vi "initialization.vi"(9 "软件版本":refnum<vi>, 10 "updateconfiguration":refnum<vi>) -> ()   [LabVIEW 2016, in "数据传输系统.lvlib"]
uses:
  <vilib>/Utility/config.llb/Read Key (String).vi
  <vilib>/Utility/config.llb/NI_LVConfig.lvlib
panel:
  in  "参数数值":T1={"CODMn"=TRUE, "CODCr"=TRUE, "DO"=TRUE, "铜"=TRUE, "PH"=TRUE, "氨氮"=TRUE, "比电导率"=TRUE, "水温"=TRUE, "COD"=TRUE, "浊度"=TRUE, "总氮"=TRUE, "总磷"=TRUE, "叶绿素a"=TRUE, "藻密度"=TRUE, "水位"=TRUE, "流速"=TRUE, "瞬时流量"=TRUE, "累积流量"=TRUE, "亚硝氮"=TRUE, "硫化物"=TRUE, "ORP"=TRUE, "铅"=TRUE, "镉"=TRUE, "锌"=TRUE, "镍"=TRUE, "锰"=TRUE, "汞"=TRUE, "气温"=TRUE, "气压"=TRUE, "风速"=TRUE, "风向"=TRUE, "盐度"=TRUE, "磷酸盐"=TRUE, "硝氮"=TRUE, "氟化物"=TRUE}
  out "配置表格":string[][](table)
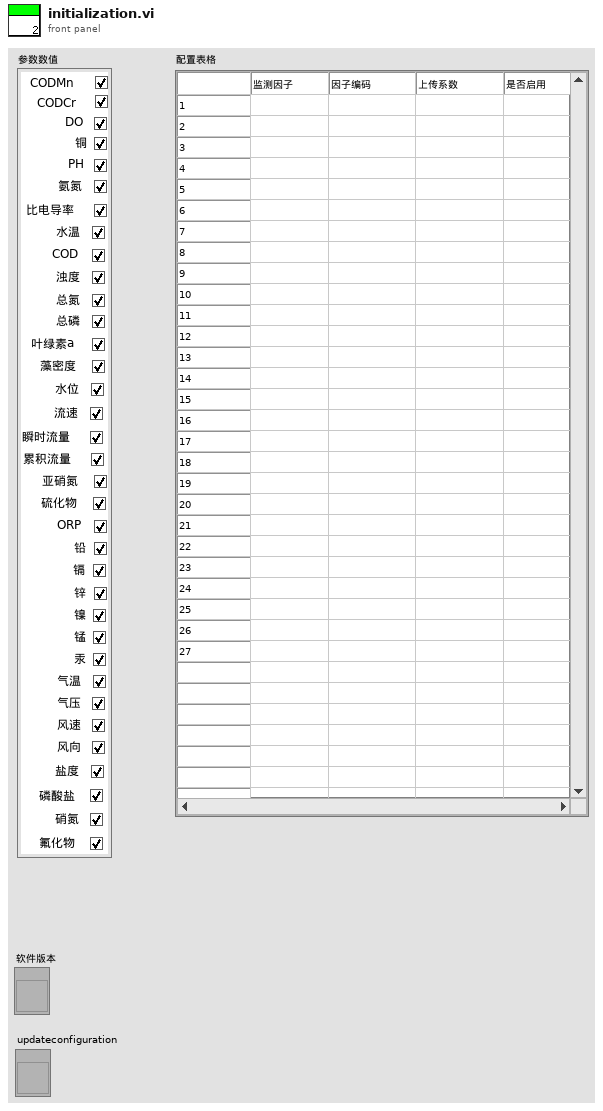
[diagram p1: front panel]
types:
  T1 = cluster{"CODMn":bool, "CODCr":bool, "DO":bool, "铜":bool, "PH":bool, "氨氮":bool, "比电导率":bool, "水温":bool, "COD":bool, "浊度":bool, "总氮":bool, "总磷":bool, "叶绿素a":bool, "藻密度":bool, "水位":bool, "流速":bool, "瞬时流量":bool, "累积流量":bool, "亚硝氮":bool, "硫化物":bool, "ORP":bool, "铅":bool, "镉":bool, "锌":bool, "镍":bool, "锰":bool, "汞":bool, "气温":bool, "气压":bool, "风速":bool, "风向":bool, "盐度":bool, "磷酸盐":bool, "硝氮":bool, "氟化物":bool}
  T2 = cluster{"setini":string, "sysini":string, "hechaini":string, "actualwrite":string, "actualread":string, "datasent":string, "反控命令信息队列":string, "反控与仪器交互":string}
  T3 = cluster{"CODMn":string, "CODCr":string, "DO":string, "铜":string, "PH":string, "氨氮":string, "比电导率":string, "水温":string, "COD":string, "浊度":string, "总氮":string, "总磷":string, "叶绿素a":string, "藻密度":string, "水位":string, "流速":string, "瞬时流量":string, "累积流量":string, "亚硝酸盐":string, "硫化物":string, "ORP":string, "铅":string, "镉":string, "锌":string, "镍":string, "锰":string, "汞":string, "气温":string, "气压":string, "风速":string, "风向":string, "盐度":string, "磷酸盐":string, "硝氮":string, "氟化物":string}
  T4 = typedef "NI_LVConfig.lvlib/Config Data RefNum.ctl" = refnum<k1>
  T5 = cluster{"[0]":string, "[1]":string, "[2]":string, "[3]":string, "[4]":string, "[5]":string, "[6]":string, "[7]":string, "[8]":string, "[9]":string, "[10]":string, "[11]":string, "[12]":string, "[13]":string, "[14]":string, "[15]":string, "[16]":string, "[17]":string, "[18]":string, "[19]":string, "[20]":string, "[21]":string, "[22]":string, "[23]":string, "[24]":string, "[25]":string, "[26]":string, "[27]":string, "[28]":string, "[29]":string, "[30]":string, "[31]":string, "[32]":string, "[33]":string, "[34]":string}
  T6 = cluster{"主机":string, "用户":string, "密码":string, "远程路径":string, "下载文件名":string, "软件版本":string}
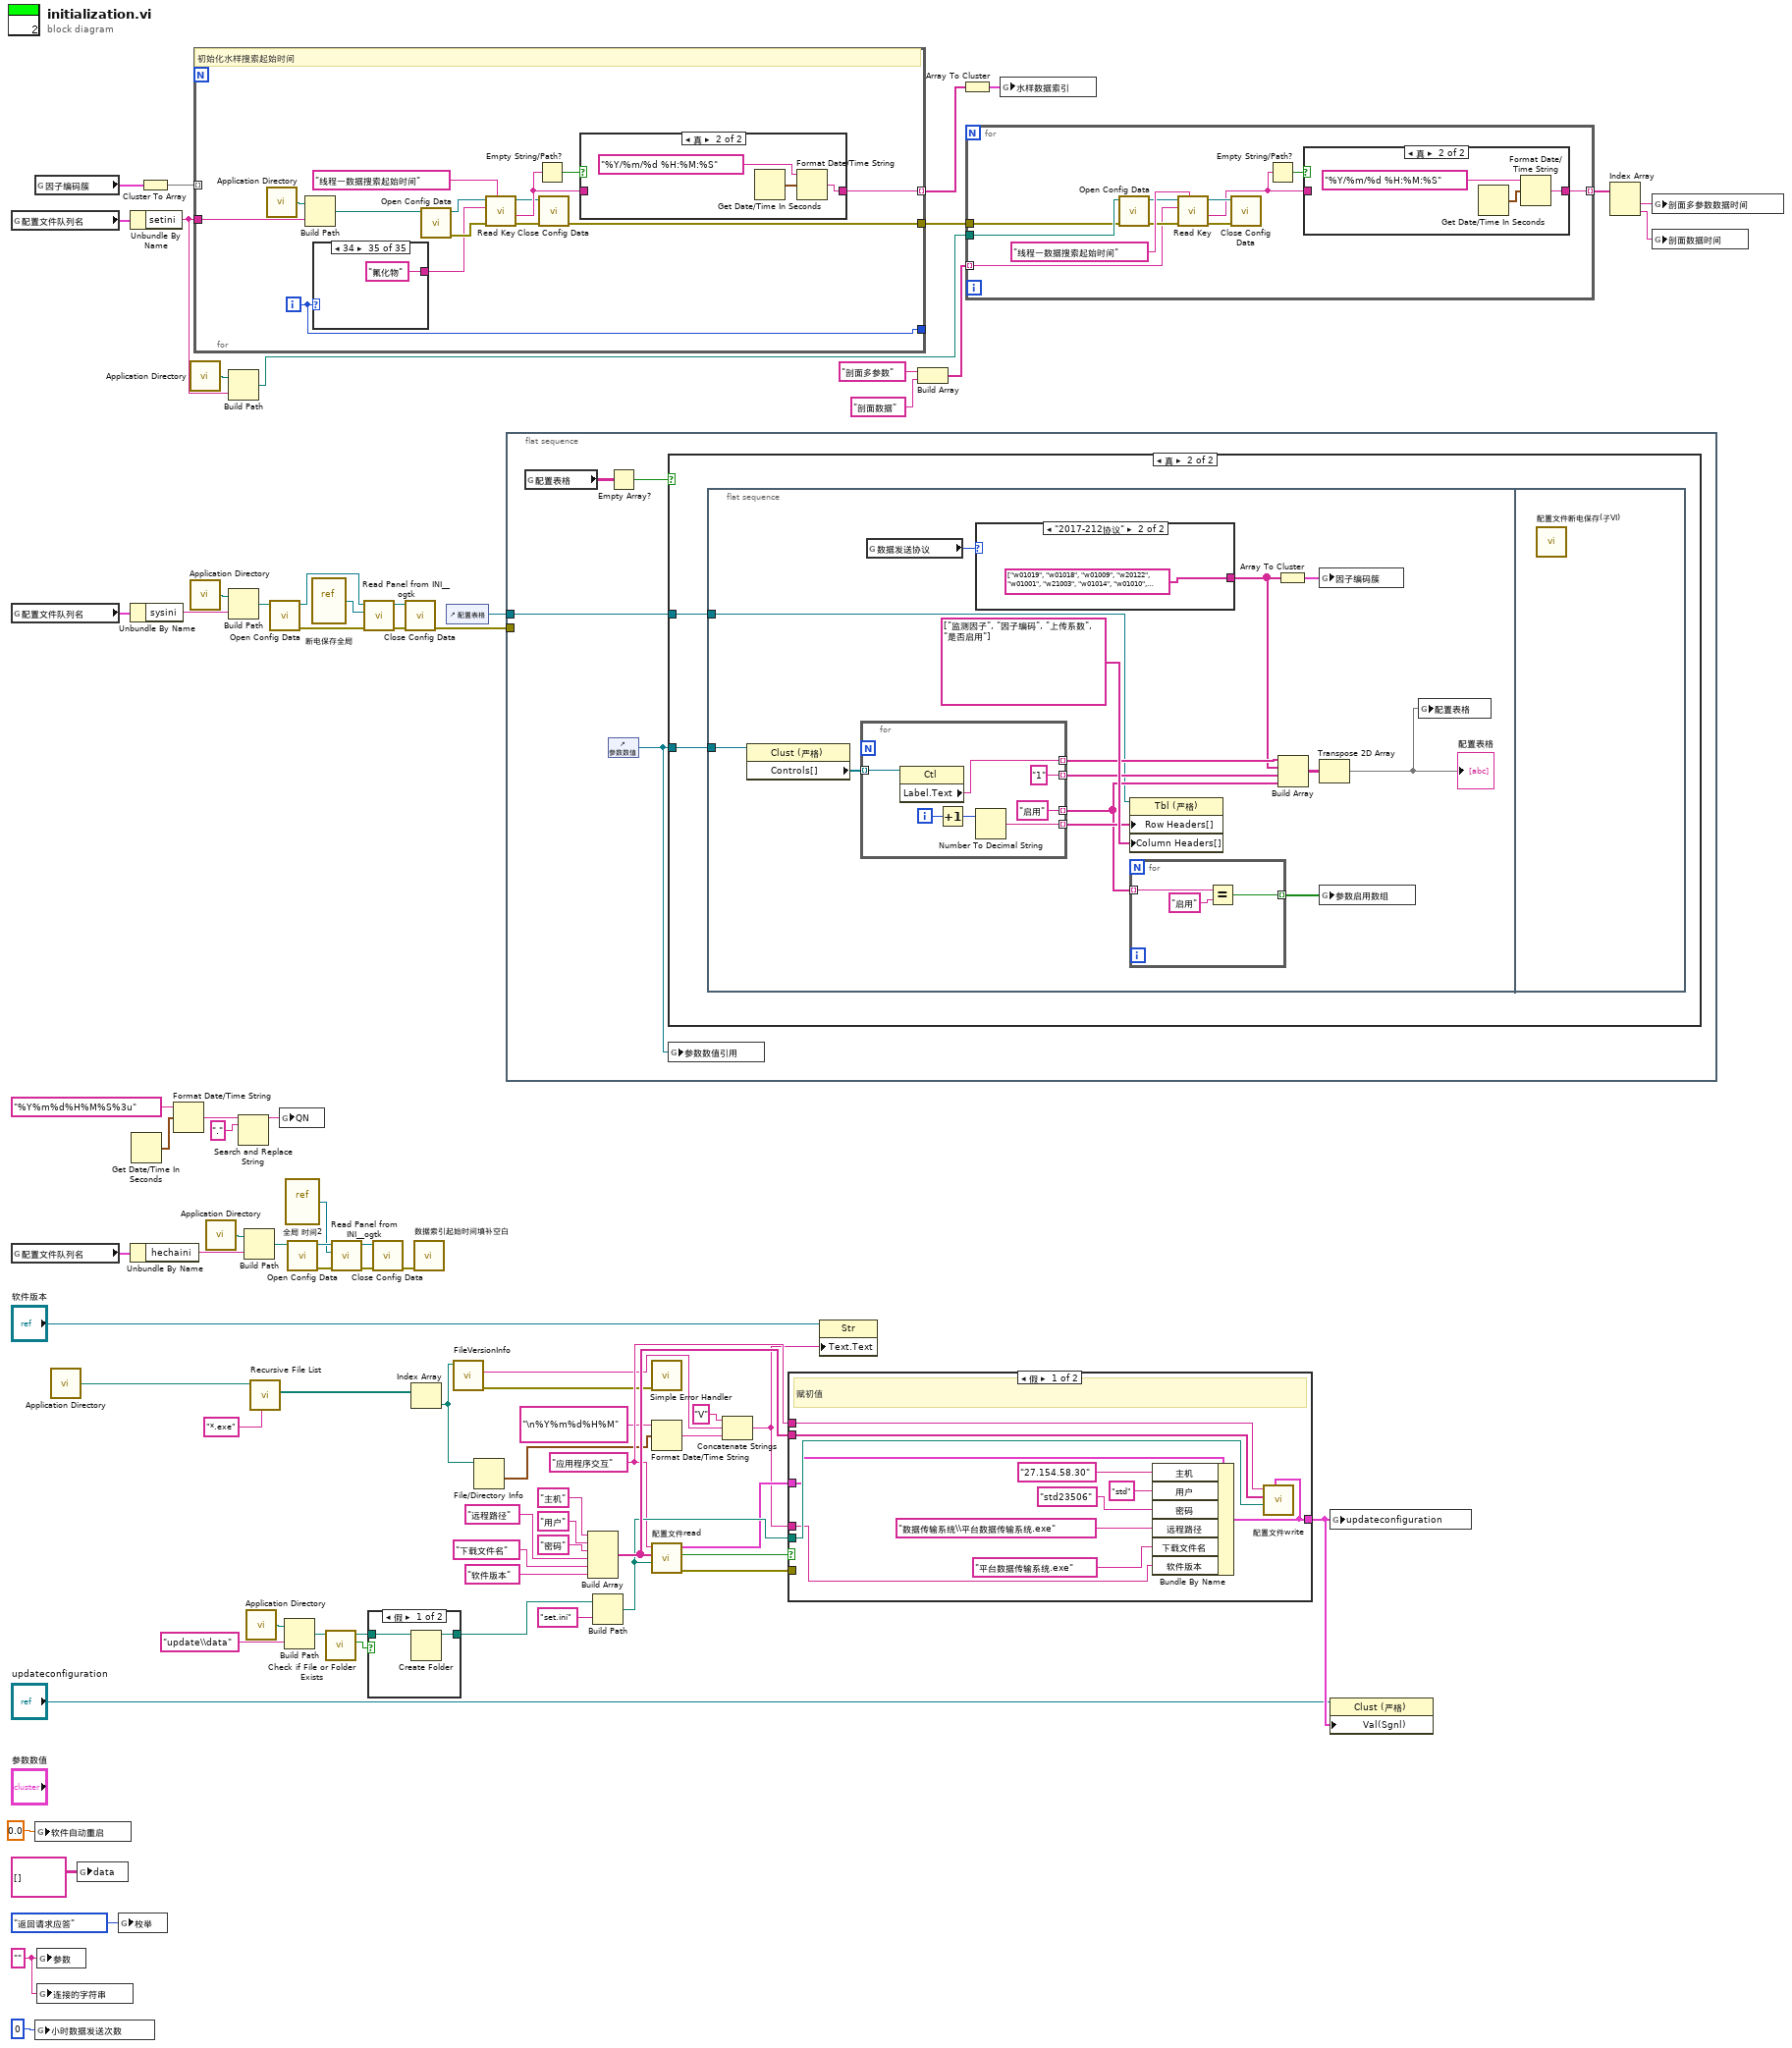
[diagram p0: block diagram]
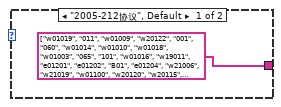
[diagram p3: hidden frame]
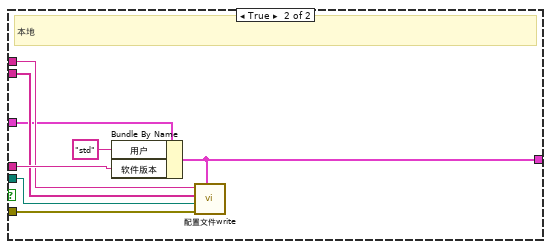
[diagram p6: hidden frame]
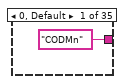
[diagram p8: hidden frame]
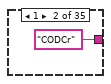
[diagram p9: hidden frame]
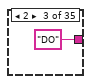
[diagram p10: hidden frame]
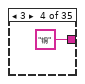
[diagram p11: hidden frame]
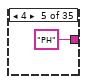
[diagram p12: hidden frame]
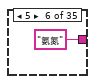
[diagram p13: hidden frame]
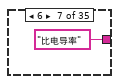
[diagram p14: hidden frame]
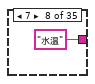
[diagram p15: hidden frame]
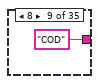
[diagram p16: hidden frame]
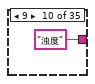
[diagram p17: hidden frame]
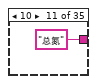
[diagram p18: hidden frame]
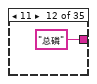
[diagram p19: hidden frame]
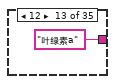
[diagram p20: hidden frame]
diagram:
  w45 = "应用程序交互" ("section")
  w6 = "" ("参数")
  n1 = global read "断电保存全局.vi" "配置文件队列名"() -> (w67:T2)
  n2 = global read "断电保存全局.vi" "配置文件队列名"() -> (w69:T2)
  n3 = global read "断电保存全局.vi" "配置文件队列名"() -> (w71:T2)
  n4 = global read "断电保存全局.vi" "因子编码簇"() -> (w65:T3)
  n5 = global write "全局1.vi" "软件自动重启"(0.0 ("软件自动重启")) -> ()
  n6 = global write "全局 小时数据发送次数.vi" "小时数据发送次数"(0 ("数值")) -> ()
  n7 = global write "全局 实时数据参数.vi" "参数"(w6) -> ()
  n8 = global write "全局 实时数据参数.vi" "连接的字符串"(w6) -> ()
  n9 = call <vilib>:"Application Directory.vi"() -> ("Application Directory"=w21:path)
  n10 = global write "全局 实时数据参数.vi" "data"(string[][] [] ("data")) -> ()
  n11 = global write "全局1.vi" "枚举"(enum16{"返回请求应答", "上传数据", "返回执行结果"}."返回请求应答" ("枚举")) -> ()
  n12 = Unbundle By Name(w67) -> ("setini"=w68:string)
  n13 = Unbundle By Name(w69) -> ("sysini"=w70:string)
  n14 = Unbundle By Name(w71) -> ("hechaini"=w72:string)
  n15 = Get Date/Time In Seconds() -> (seconds since 1Jan1904=w10:timestamp)
  n16 = Cluster To Array(cluster=w65) -> (array=w40:string[])
  n17 = Format Date/Time String(time format string (%c)="%Y%m%d%H%M%S%3u" ("时间格式字符串(%c)"), seconds (now)=w10) -> (date/time string=w11:string)  [unwired: 1 in]
  n18 = call <vilib>:"Application Directory.vi"() -> ("Application Directory"=w61:path)
  n19 = call <vilib>:"Application Directory.vi"() -> ("Application Directory"=w27:path)
  n20 = for {
    tunnel: w40 -> [_] mode=indexing
    tunnel: [w85] -> _
    tunnel: [w82] -> w41 mode=indexing
    tunnel: [w81] -> w63
    tunnel: w68 -> [w80]
    i -> [w85]
    # "初始化水样搜索起始时间"
    n21 = call <vilib>:"Application Directory.vi"() -> ("Application Directory"=w93:path)
    n22 = Build Path(base path=w93, name or relative path=w80) -> (appended path=w92:path)
    n23 = case shown="34" w85 {
      tunnel: ["CODMn" "CODCr" "DO" "铜" "PH" "氨氮" "比电导率" "水温" "COD" "浊度" "总氮" "总磷" "叶绿素a" "藻密度" "水位" "流速" "瞬时流量" "累积流量" "亚硝氮" "硫化物" "ORP" "铅" "镉" "锌" "镍" "锰" "汞" "气温" "气压" "风速" "风向" "盐度" "磷酸盐" "硝氮" "氟化物"] -> w88
      frame 0, Default {
      }
      frame 1 {
      }
      frame 2 {
      }
      frame 3 {
      }
      frame 4 {
      }
      frame 5 {
      }
      frame 6 {
      }
      frame 7 {
      }
      frame 8 {
      }
      frame 9 {
      }
      frame 10 {
      }
      frame 11 {
      }
      frame 12 {
      }
      frame 13 {
      }
      frame 14 {
      }
      frame 15 {
      }
      frame 16 {
      }
      frame 17 {
      }
      frame 18 {
      }
      frame 19 {
      }
      frame 20 {
      }
      frame 21 {
      }
      frame 22 {
      }
      frame 23 {
      }
      frame 24 {
      }
      frame 25 {
      }
      frame 26 {
      }
      frame 27 {
      }
      frame 28 {
      }
      frame 29 {
      }
      frame 30 {
      }
      frame 31 {
      }
      frame 32 {
      }
      frame 33 {
      }
      frame 34 {
      }
    }
    n24 = call <vilib>:"Open Config Data.vi"("configuration file path"=w92) -> ("error out"=w90:errorcluster, "refnum"=w91:T4)  [unwired: 8 in, 1 out]
    n25 = call-poly <vilib>:"Read Key.vi"("section"="线程一数据搜索起始时间", "error in (no error)"=w90, "key"=w88, "refnum"=w91) -> ("error out"=w83:errorcluster, "value"=w86:string, "refnum out"=w84:T4)  [unwired: 4 in, 1 out]
    n26 = Empty String/Path?(string/path=w86) -> (empty?=w87:bool)
    n27 = call <vilib>:"Close Config Data.vi"("error in (no error)"=w83, "refnum"=w84) -> ("error out"=w81:errorcluster)  [unwired: 8 in, 1 out]
    n28 = case shown="真" w87 {
      tunnel: [w94 w95] -> w82
      tunnel: w86 -> [w94 _]
      frame False {
      }
      frame True {
        n29 = Get Date/Time In Seconds() -> (seconds since 1Jan1904=w97:timestamp)
        n30 = Format Date/Time String(time format string (%c)="%Y/%m/%d %H:%M:%S" ("时间格式字符串(%c)"), seconds (now)=w97) -> (date/time string=w95:string)  [unwired: 1 in]
      }
    }
  }
  n31 = call <vilib>:"Application Directory.vi"() -> ("Application Directory"=w33:path)
  n32 = Build Path(base path=w61, name or relative path=w68) -> (appended path=w62:path)
  n33 = Build Path(base path=w27, name or relative path=w70) -> (appended path=w28:path)
  n34 = Search and Replace String(input string=w11, search string="." ("搜索字符串")) -> (result string=w13:string)  [unwired: 6 in, 3 out]
  n35 = Build Path(base path=w33, name or relative path=w72) -> (appended path=w32:path)
  n36 = call <vilib>:"Application Directory.vi"() -> ("Application Directory"=w58:path)
  n37 = call <vilib>:"Recursive File List.vi"("pattern"="*.exe", "Folder Path"=w21) -> ("All Files in Dir"=w15:path[])  [unwired: 5 in, 4 out]
  n38 = call <vilib>:"Open Config Data.vi"("configuration file path"=w28) -> ("error out"=w23:errorcluster, "refnum"=w24:T4)  [unwired: 8 in, 1 out]
  n39 = global write "全局1.vi" "QN"(w13) -> ()
  n40 = Build Path(base path=w58, name or relative path="update\\data" ("名称或相对路径")) -> (appended path=w57:path)
  n41 = vi-ref "全局 时间2.vi"() -> (w35:refnum<vi>)
  n42 = call <vilib>:"Open Config Data.vi"("configuration file path"=w32) -> ("error out"=w37:errorcluster, "refnum"=w36:T4)  [unwired: 8 in, 1 out]
  n43 = vi-ref "断电保存全局.vi"() -> (w25:refnum<vi>)
  n44 = call <vilib>:"Check if File or Folder Exists.vi"("path"=w57) -> ("file or folder exists?"=w56:bool, "dup path"=w55:path)  [unwired: 8 in, 1 out]
  n45 = call <userlib>:"Read Panel from INI__ogtk.vi"("error in (no error)"=w37, "VI ref"=w35, "refnum"=w36) -> ("error out"=w38:errorcluster, "refnum out"=w34:T4)  [unwired: 7 in]
  n46 = call <userlib>:"Read Panel from INI__ogtk.vi"("error in (no error)"=w23, "VI ref"=w25, "refnum"=w24) -> ("error out"=w29:errorcluster, "refnum out"=w26:T4)  [unwired: 7 in]
  n47 = case shown="假" w56 {
    tunnel: w55 -> [w134 w135]
    tunnel: [w133 w135] -> w60
    frame False {
      n48 = Create Folder(path (use dialog)=w134) -> (created path=w133:path)  [unwired: 2 in, 2 out]
    }
    frame True {
    }
  }
  n49 = call <vilib>:"Close Config Data.vi"("error in (no error)"=w38, "refnum"=w34) -> ("error out"=w39:errorcluster)  [unwired: 8 in, 1 out]
  n50 = call <vilib>:"Close Config Data.vi"("error in (no error)"=w29, "refnum"=w26) -> ("error out"=w64:errorcluster)  [unwired: 8 in, 1 out]
  n51 = Index Array(array=w15) -> (element=w16:path)  [unwired: 1 in]
  n52 = call "数据索引起始时间填补空白.vi"("error in (no error)"=w39) -> ()  [unwired: 10 in, 1 out]
  n53 = control-ref of="配置表格"() -> (w3:refnum<vi>)
  n54 = call <vilib>:"FileVersionInfo.vi"("Application Path in"=w16) -> ("error out"=w22:errorcluster, "File Version Info"=w31:string)  [unwired: 7 in, 2 out]
  n55 = File/Directory Info(path=w16) -> (last mod=w17:timestamp)  [unwired: 1 in, 6 out]
  n56 = flat-sequence {
    tunnel: w64 -> [_]
    tunnel: w3 -> [w137]
    frame #0 {
      n57 = global read "断电保存全局.vi" "配置表格"() -> (w139:string[][])
      n58 = Empty Array?(array=w139) -> (empty?=w138:bool)
      n59 = control-ref of="参数数值"() -> (w136:refnum<vi>)
      n60 = case shown="真" w138 {
        tunnel: w137 -> [_ w141]
        tunnel: w136 -> [_ w140]
        frame False {
        }
        frame True {
          n61 = flat-sequence {
            tunnel: w141 -> [w143]
            tunnel: w140 -> [w142]
            frame #0 {
              n62 = property on="属性节点" class="Clust (严格)"(reference=w142) -> ("Controls[]"=w151:refnum<vi>[])  [unwired: 1 in, 2 out]
              n63 = for {
                tunnel: w151 -> [w167] mode=indexing
                tunnel: [w166] -> w153 mode=indexing
                tunnel: [w164] -> w152 mode=indexing
                tunnel: ["1"] -> w146 mode=indexing
                tunnel: ["启用"] -> w145 mode=indexing
                i -> [w165]
                n64 = property class="Ctl"(reference=w167) -> ("Label.Text"=w166:string)  [unwired: 1 in, 2 out]
                n65 = Increment(x=w165) -> (x+1=w163:i32)
                n66 = Number To Decimal String(number=w163) -> (decimal integer string=w164:string)  [unwired: 1 in]
              }
              n67 = global read "断电保存全局.vi" "数据发送协议"() -> (w149:enum16{"2005-212协议", "2017-212协议"})
              n68 = case shown="\"2017-212协议\"" w149 {
                tunnel: [string[] ["w01019", "011", "w01009", "w20122", "001", "060", "w01014", "w01010", "w01018", "w01003", "065", "101", "w01016", "w19011", "e01201", "e01202", "B01", "e01204", "w21006", "w21019", "w01100", "w20120", "w20115", "w20123", "w20121", "w20124", "w20111", "a01001", "a01006", "a01007", "a01008", "w01002", "w21015", "w21007", "w21017"] string[] ["w01019", "w01018", "w01009", "w20122", "w01001", "w21003", "w01014", "w01010", "w01018", "w01003", "w21001", "w21011", "w01016", "w19011", "e01201", "e01202", "e01203", "e01204", "w21006", "w21019", "w01100", "w20120", "w20115", "w20123", "w20121", "w20124", "w20111", "a01001", "a01006", "a01007", "a01008", "w01002", "w21015", "w21007", "w21017"]] -> w147
                frame "2005-212协议", Default {
                }
                frame "2017-212协议" {
                }
              }
              n69 = property on="属性节点" class="Tbl (严格)"(reference=w143, "Row Headers[]"=w152, "Column Headers[]"=string[] ["监测因子", "因子编码", "上传系数", "是否启用"]) -> ()  [unwired: 1 in, 2 out]
              n70 = for {
                tunnel: w145 -> [w158] mode=indexing
                tunnel: [w156] -> w144 mode=indexing
                n71 = Equal?(x=w158, y="启用") -> (x = y?=w156:bool)
              }
              n72 = Array To Cluster(array=w147) -> (cluster=w148:T5)
              n73 = Build Array(w153, w147, w146, w145) -> (w155:string[][])
              n74 = global write "断电保存全局.vi" "因子编码簇"(w148) -> ()
              n75 = Transpose 2D Array(2D array=w155) -> (transposed array=w150:string[][])
              "配置表格" <- w150
              n76 = global write "断电保存全局.vi" "参数启用数组"(w144) -> ()
              n77 = global write "断电保存全局.vi" "配置表格"(w150) -> ()
            }
            frame #1 {
              n78 = call "配置文件断电保存(子VI).vi"() -> ()  [unwired: 12 in]
            }
          }
        }
      }
      n79 = global write "断电保存全局.vi" "参数数值引用"(w136) -> ()
    }
  }
  n80 = Build Array("主机" ("section"), "用户" ("section"), "密码" ("key"), "远程路径" ("key"), "下载文件名" ("key"), "软件版本" ("key")) -> (w54:string[])
  n81 = Build Path(base path=w60, name or relative path="set.ini" ("名称或相对路径")) -> (appended path=w46:path)
  n82 = call <vilib>:"Simple Error Handler.vi"("error in (no error)"=w22) -> ()  [unwired: 4 in, 5 out]
  n83 = Format Date/Time String(time format string (%c)="\n%Y%m%d%H%M" ("时间格式字符串(%c)"), seconds (now)=w17) -> (date/time string=w20:string)  [unwired: 1 in]
  n84 = call "配置文件read.vi"("configuration file path"=w46, "键数组"=w54, "段"=w45) -> ("error out"=w47:errorcluster, "section exists?"=w43:bool, "updateconfiguration"=w44:T6)  [unwired: 6 in]
  n85 = Concatenate Strings("V" ("字符串"), w31, w20) -> (w1:string)
  n86 = case shown="假" w43 {
    tunnel: w44 -> [w174 w181]
    tunnel: [w173 w180] -> w73
    tunnel: w1 -> [w168 w186]
    tunnel: w45 -> [w177 w185]
    tunnel: w54 -> [w176 w184]
    tunnel: w46 -> [w175 w183]
    tunnel: w47 -> [_ w182]
    frame False {
      # "赋初值"
      n87 = Bundle By Name(cluster=w174, "主机"="27.154.58.30" ("key"), "用户"="std", "密码"="std23506", "远程路径"="数据传输系统\\平台数据传输系统.exe", "下载文件名"="平台数据传输系统.exe", "软件版本"=w168) -> (w173:T6)
      n88 = call "配置文件write.vi"("updateconfiguration"=w173, "configuration file path"=w175, "键数组"=w176, "段"=w177) -> ()  [unwired: 7 in, 1 out]
    }
    frame True {
      # "本地"
      n89 = Bundle By Name(cluster=w181, "用户"="std", "软件版本"=w186) -> (w180:T6)
      n90 = call "配置文件write.vi"("updateconfiguration"=w180, "error in (no error)"=w182, "configuration file path"=w183, "键数组"=w184, "段"=w185) -> ()  [unwired: 6 in, 1 out]
    }
  }
  n91 = property class="Str"(reference="软件版本", "Text.Text"=w1) -> ()  [unwired: 1 in, 2 out]
  n92 = Build Array("剖面多参数" ("key"), "剖面数据" ("key")) -> (w76:string[])
  n93 = Array To Cluster(array=w41) -> (cluster=w42:T5)
  n94 = for {
    tunnel: w62 -> [w197]
    tunnel: w63 -> [w196]
    tunnel: w76 -> [w188] mode=indexing
    tunnel: [w187] -> w77 mode=indexing
    n95 = call <vilib>:"Open Config Data.vi"("error in (no error)"=w196, "configuration file path"=w197) -> ("error out"=w193:errorcluster, "refnum"=w194:T4)  [unwired: 7 in, 1 out]
    n96 = call-poly <vilib>:"Read Key.vi"("section"="线程一数据搜索起始时间", "error in (no error)"=w193, "key"=w188, "refnum"=w194) -> ("error out"=w191:errorcluster, "value"=w190:string, "refnum out"=w192:T4)  [unwired: 4 in, 1 out]
    n97 = call <vilib>:"Close Config Data.vi"("error in (no error)"=w191, "refnum"=w192) -> ()  [unwired: 8 in, 2 out]
    n98 = Empty String/Path?(string/path=w190) -> (empty?=w189:bool)
    n99 = case shown="真" w189 {
      tunnel: [w198 w199] -> w187
      tunnel: w190 -> [w198 _]
      frame False {
      }
      frame True {
        n100 = Get Date/Time In Seconds() -> (seconds since 1Jan1904=w201:timestamp)
        n101 = Format Date/Time String(time format string (%c)="%Y/%m/%d %H:%M:%S" ("时间格式字符串(%c)"), seconds (now)=w201) -> (date/time string=w199:string)  [unwired: 1 in]
      }
    }
  }
  n102 = global write "全局 水样时间.vi" "水样数据索引"(w42) -> ()
  n103 = global write "update全局.vi" "updateconfiguration"(w73) -> ()
  n104 = property on="属性节点" class="Clust (严格)"(reference="updateconfiguration", "Val(Sgnl)"=w73) -> ()  [unwired: 1 in, 2 out]
  n105 = Index Array(array=w77) -> (element #1=w78:string, element #2=w79:string)  [unwired: 2 in]
  n106 = global write "全局 水样时间.vi" "剖面多参数数据时间"(w78) -> ()
  n107 = global write "全局 水样时间.vi" "剖面数据时间"(w79) -> ()
